vi "Broken Rotor Bar Harmonics (1 Motor).vi"(0 "spectrum information":T2={"spectrum"={"f0"=0.0, "df"=0.1, "magnitude [dB]"=[]}, "demodulated? (F)"=FALSE}, 1 "fundamental frequency [Hz]":dbl=50.0, 5 "slip":dbl, 7 "max sideband order (10)":u8=10, 11 "error in (no error)":errorcluster) -> (4 "upper sidebands":T1, 6 "lower sidebands":T1, 8 "max sideband magnitude [dB]":dbl, 15 "error out":errorcluster)   [LabVIEW 2014, in "NI_EP_Motor Monitoring.lvlib"]
doc: "Calculates the sideband harmonics to detect broken rotor bars. You must manually select the polymorphic instance you want to use."
uses:
  <vilib>/addons/Electrical Power/Motor Monitoring/NI_EP_Motor Monitoring.lvlib
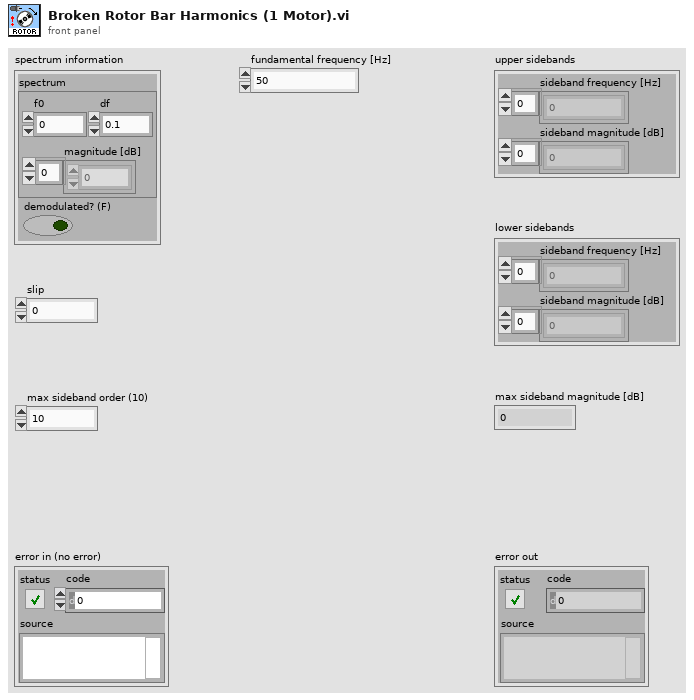
[diagram p1: front panel]
types:
  T1 = cluster{"sideband frequency [Hz]":dbl[], "sideband magnitude [dB]":dbl[]}
  T2 = cluster{"spectrum":cluster{"f0":dbl, "df":dbl, "magnitude [dB]":dbl[]}, "demodulated? (F)":bool}
  T3 = cluster{"f0":dbl, "df":dbl, "magnitude [dB]":dbl[]}
  T4 = cluster{"frequency [Hz]":dbl[], "magnitude [dB]":dbl[]}
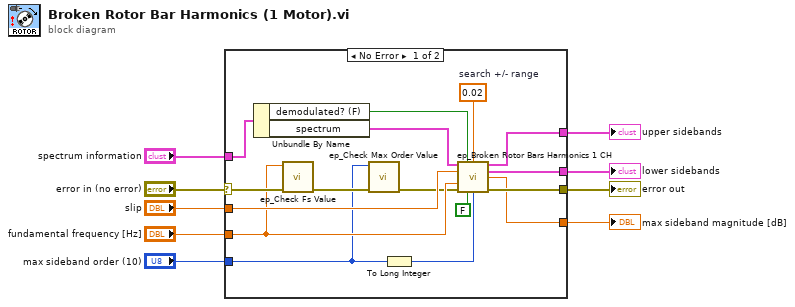
[diagram p0: block diagram]
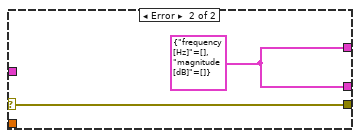
[diagram p2: hidden frame]
diagram:
  n1 = case shown="No Error" "error in (no error)" {
    selector: "error in (no error)" -> [w14 w27]
    tunnel: "spectrum information" -> [w24 _]
    tunnel: "fundamental frequency [Hz]" -> [w13 _]
    tunnel: [w25 w27] -> w6
    tunnel: [w20 w26] -> w5
    tunnel: [w19 w26] -> w4
    tunnel: "slip" -> [w16 _]
    tunnel: "max sideband order (10)" -> [w10 _]
    tunnel: [w15 _] -> w1
    frame No Error {
      w21 = 0.02  # search +/- range
      n2 = Unbundle By Name(w24) -> ("demodulated? (F)"=w22:bool, "spectrum"=w23:T3)
      n3 = call <vilib>:"ep_Check Fs Value.vi"("error in (no error)"=w14, "fundamental frequency [Hz]"=w13) -> ("error out"=w12:errorcluster)  [unwired: 9 in]
      n4 = call <vilib>:"ep_Check Max Order Value.vi"("error in (no error)"=w12, "max sideband order"=w10) -> ("error out"=w11:errorcluster)  [unwired: 9 in]
      n5 = To Long Integer(number=w10) -> (32bit integer=w17:i32)
      n6 = call <vilib>:"ep_Broken Rotor Bars Harmonics 1 CH.vi"("spectra"=w23, "demodulated? (F)"=w22, "search +/- percentage"=w21, "slip"=w16, "fundamental frequency [Hz]"=w13, "error in (no error)"=w11, "sinc interpolation? (F)"=FALSE, "max sideband order"=w17) -> ("upper sidebands"=w20:T4, "lower sidebands"=w19:T4, "max sideband magnitude [dB]"=w15:dbl, "error out"=w25:errorcluster)  [unwired: 4 in]
    }
    frame Error {
      w26 = T4 {"frequency [Hz]"=[], "magnitude [dB]"=[]} ("upper sidebands")
    }
  }
  "error out" <- w6
  "upper sidebands" <- w5
  "lower sidebands" <- w4
  "max sideband magnitude [dB]" <- w1
